vi "onDisconnection.vi"(8 "error in (no error)":errorcluster, 11 "Connection.TCP-TLS in":refnum<class "Connection.TCP-TLS.lvclass">) -> (0 "error out":errorcluster, 3 "No Connection":refnum<class "Connection.TCP-TLS.lvclass">)   [LabVIEW 2020, in "Connection.TCP-TLS.lvclass"]
uses:
  Connection.TCP-TLS.lvclass
  Connection.TCP-TLS.lvclass/Connection.TCP-TLS.ctl
  <vilib>/LabVIEW Open Source Project/MQTT TCP Connection/MQTT_TCP/Connection/TCPConnection.lvclass
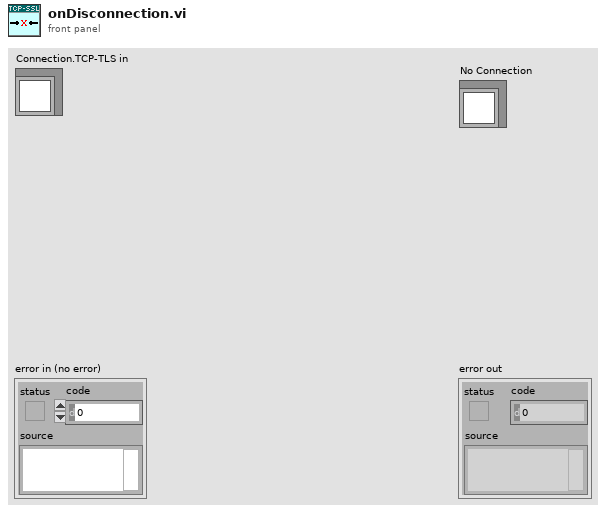
[diagram p1: front panel]
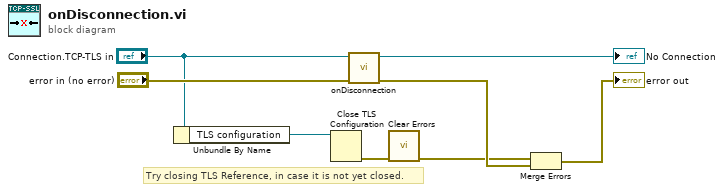
[diagram p0: block diagram]
diagram:
  # "Try closing TLS Reference, in case it is not yet closed."
  n1 = Unbundle By Name("Connection.TCP-TLS in") -> ("TLS configuration"=w6:refnum<k36>)
  n2 = Close TLS Configuration(11:w6) -> (0:w5:errorcluster)  [unwired: 1 in]
  n3 = call-parent "onDisconnection.vi"("error in (no error)"="error in (no error)", "TCPConnection in"="Connection.TCP-TLS in") -> ("error out"=w2:errorcluster, "No Connection"=→"No Connection":refnum<class "Connection.TCP-TLS.lvclass">)  [unwired: 8 in]
  n4 = call <vilib>:"Clear Errors.vi"("error in (no error)"=w5) -> ("error out"=w1:errorcluster)  [unwired: 5 in, 1 out]
  n5 = Merge Errors(w1, w2) -> (→"error out":errorcluster)
